vi "GetTorque(mNm).vi"(8 "error in (no error)":errorcluster, 11 "Motor Base in":refnum<class "Motor Base.lvclass">) -> (0 "error out":errorcluster, 2 "torque(mNm)":dbl, 3 "Motor Base out":refnum<class "Motor Base.lvclass">)   [LabVIEW 2016, in "Motor Base.lvlib" / "Motor Base.lvclass"]
uses:
  Motor Base.lvclass
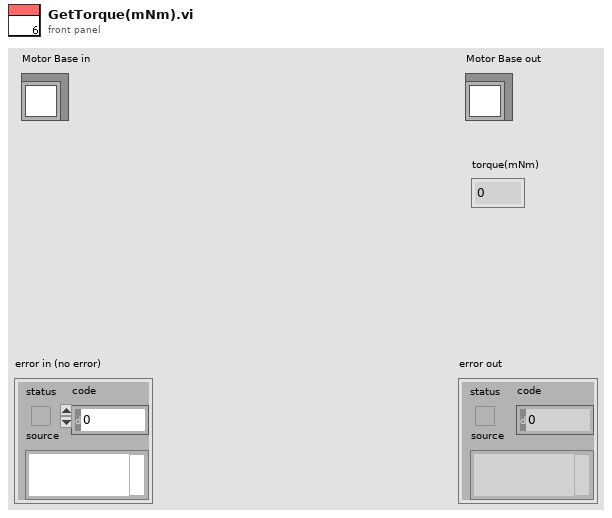
[diagram p1: front panel]
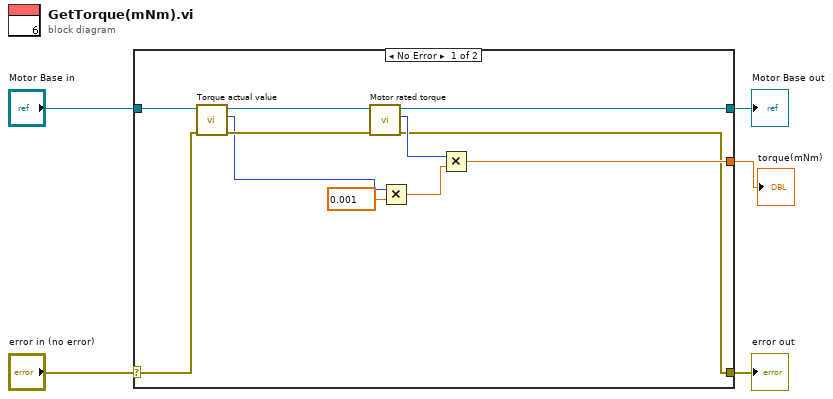
[diagram p0: block diagram]
diagram:
  n1 = case shown="No Error" "error in (no error)" {
    selector: "error in (no error)" -> [w14 w18]
    tunnel: [w7 w18] -> w4
    tunnel: [w9 w17] -> w2
    tunnel: "Motor Base in" -> [w16 w17]
    tunnel: [w8 _] -> w1
    frame No Error {
      n2 = call-dynamic "Torque actual value.vi"("error in"=w14, "Motor Base in"=w16) -> ("error out"=w13:errorcluster, "Data"=w6:i16, "Motor Base out"=w15:refnum<class "Motor Base.lvclass">)  [unwired: 7 in]
      n3 = call-dynamic "Motor rated torque.vi"("error in"=w13, "Motor Base in"=w15) -> ("error out"=w7:errorcluster, "Data"=w11:u32, "Motor Base out"=w9:refnum<class "Motor Base.lvclass">)  [unwired: 7 in]
      n4 = Multiply(x=w6, y=0.001) -> (x*y=w10:dbl)
      n5 = Multiply(x=w11, y=w10) -> (x*y=w8:dbl)
    }
    frame Error {
    }
  }
  "error out" <- w4
  "Motor Base out" <- w2
  "torque(mNm)" <- w1
